vi "Choreo_DifferentialSample_GetTypeName.vi"() -> (3 "TypeName":string="DifferentialSample")   [LabVIEW 2019, in "ChoreoLib.lvlib"]
doc: "Return the type name of this sample. The response string is \"DifferentialSample\".\n\nInputs:\n -- None --\n\nOutputs:\n -- TypeName - string - Returned name of this type of trajectory sample."
uses:
  ChoreoLib.lvlib
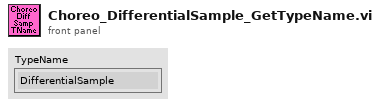
[diagram p1: front panel]
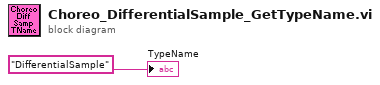
[diagram p0: block diagram]
diagram:
  "TypeName" <- "DifferentialSample"
